vi "Get Harmonic.vi"(8 "error in (no error)":errorcluster, 11 "VISA resource name":refnum<visa-resource-name>) -> (0 "error out":errorcluster, 1 "Fundamental":u16, 2 "Harmonic Value":i32, 3 "VISA resource name out":refnum<visa-resource-name>)   [LabVIEW 2014, in "Fluke 5XXX Series Multicalibrators.lvlib"]
doc: "Returns the present instrument harmonic characteristic and location of the fundamental output Primary (the NORMAL terminals) or Secondary (the AUX terminals).\n\nNote:\n\nThis VI is available only for instrument models 5500A and 5520A."
uses:
  Fluke 5XXX Series Multicalibrators.lvlib
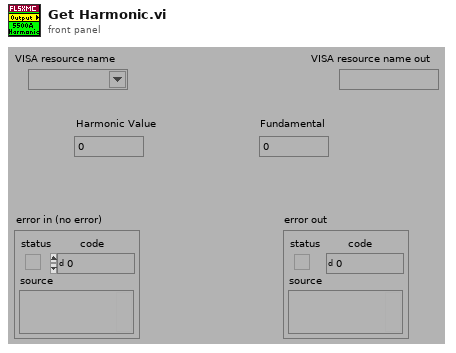
[diagram p1: front panel]
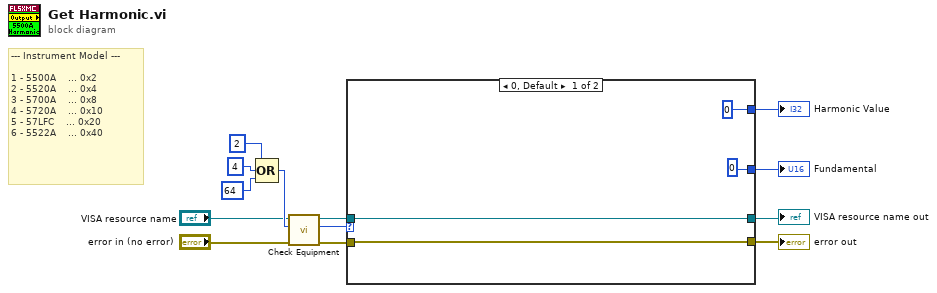
[diagram p0: block diagram]
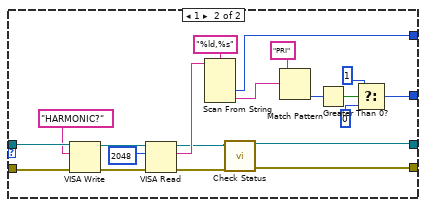
[diagram p2: hidden frame]
diagram:
  # "--- Instrument Model ---\n\n1 - 5500A    ... 0x2\n2 - 5520A    ... 0x4\n3 - 5700A    ... 0x8\n4 - 5720A    ... 0x10\n5 - 57LFC    ... 0x20\n6 - 5522A    ... 0x40"
  n1 = Compound Arithmetic op=OR(2 ("Numeric"), 4 ("Numeric"), 64 ("Numeric")) -> (w10:i32)
  n2 = call "Check Equipment.vi"("error in (no error)"="error in (no error)", "Bit Mask"=w10, "VISA resource name"="VISA resource name") -> ("error out"=w13:errorcluster, "Present?"=w12:u32, "VISA resource name out"=w11:refnum<visa-resource-name>)  [unwired: 6 in]
  n3 = case shown="0, Default" w12 {
    tunnel: [w16 w36] -> w7
    tunnel: w13 -> [w17 w35]
    tunnel: w11 -> [w16 w34]
    tunnel: [w17 w37] -> w8
    tunnel: [0 w25] -> w3
    tunnel: [u16 0 ("f") w19] -> w4
    frame 0, Default {
    }
    frame 1 {
      n4 = VISA Write(VISA resource name=w34, write buffer="HARMONIC?", error in (no error)=w35) -> (VISA resource name out=w31:refnum<visa-resource-name>, error out=w30:errorcluster)  [unwired: 1 out]
      n5 = VISA Read(VISA resource name=w31, byte count=u32 2048 ("byte count (0)"), error in (no error)=w30) -> (VISA resource name out=w26:refnum<visa-resource-name>, read buffer=w27:string, error out=w28:errorcluster)  [unwired: 1 out]
      n6 = Scan From String(format string="%ld,%s", input string=w27) -> (output 1=w25:i32, output 2=w24:string)  [unwired: 4 in, 3 out]
      n7 = call "Check Status.vi"("VISA resource name"=w26, "error in (no error)"=w28) -> ("VISA resource name out"=w36:refnum<visa-resource-name>, "error out"=w37:errorcluster)  [unwired: 12 in]
      n8 = Match Pattern(string=w24, regular expression="PRI") -> (offset past match=w22:i32)  [unwired: 1 in, 3 out]
      n9 = Greater Than 0?(x=w22) -> (x > 0?=w18:bool)
      n10 = Select(t=u16 1 ("f"), s=w18, f=u16 0) -> (s? t:f=w19:u16)
    }
  }
  "Harmonic Value" <- w3
  "Fundamental" <- w4
  "VISA resource name out" <- w7
  "error out" <- w8
